vi "PublishToTopic.vi"() -> ()   [LabVIEW 2016]
uses:
  ROS/Code/Console/Servers/ServerSubs/TopicDef.ctl
  ROS/Code/SubVIs/_ROSDirection.ctl
  ROS/MessageBuilding/std_msgs/subs/stringScalar.vi
panel:
  in  "String":string
  in  "Stop Button":bool
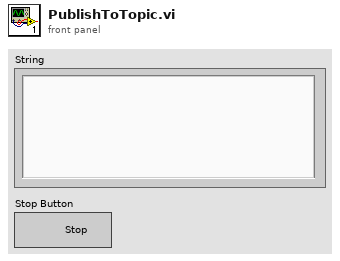
[diagram p1: front panel]
types:
  T1 = typedef "TopicDef.ctl" = cluster{"Topic":string, "Type":string, "Action":T2, "Update (ms)":u16, "queue size":u16}
  T2 = typedef "_ROSDirection.ctl" = enum16{"Node", "Publisher", "Subscriber", "ServiceClient", "ServiceProvider"}
  T3 = typedef "_ROSControl.ctl" = cluster{"topic port":u16, "Node":string, "topic":string, "type":string, "node port":u16, "error ":errorcluster, "Direction":T2, "Update (ms)":u16, "FIFO size":u16}
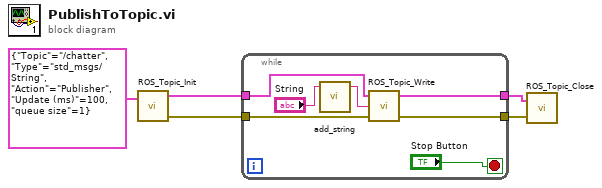
[diagram p0: block diagram]
diagram:
  n1 = call "ROS_Topic_Init.vi"("Definitions"=T1 {"Topic"="/chatter", "Type"="std_msgs/String", "Action"=enum."Publisher", "Update (ms)"=100, "queue size"=1}) -> ("ROS out"=w4:T3, "error out"=w3:errorcluster)  [unwired: 2 in]
  n2 = while {
    tunnel: w4 -> [w12]
    tunnel: w3 -> [w10]
    tunnel: [w9] -> w2
    tunnel: [w8] -> w1
    stop <- "Stop Button" stop-if-true
    n3 = call-poly "add_string.vi"("msg in"="String") -> ("msg out"=w11:string)  [unwired: 4 in]
    n4 = call "ROS_Topic_Write.vi"("error in (no error)"=w10, "Msg in"=w11, "ROS in"=w12) -> ("error out"=w8:errorcluster, "ROS out"=w9:T3)  [unwired: 1 in]
  }
  n5 = call "ROS_Topic_Close.vi"("error in"=w1, "ROS in"=w2) -> ()  [unwired: 2 in, 1 out]
